vi "Host_Model_Updating.vi"(11 "Setup Parameters and Controls":T3={"Modeling Parameters input controls"={"beam_length"=0.3525, "youngs_modulus"=209500000000.0, "torsion_spring"=0.0, "beam_height"=0.00635, "beam_width"=0.0508, "beam_density"=7900.0, "number_of_FEA_nodes"=40, "accelerometer_mass"=0.055}, "Mockbear input controls"={"Dataset"="test7", "Resample Method"=enum."Auto Resample"}, "Simulation Parameters input controls"={"Eigensolver "=enum."LEMP", "Models Forcasted"=5, "Max Roller Velocity"=3.32, "Max Roller Position Percent"=0.43, "Min Roller Position Percent"=0.155}, "Program Controls"={"Frequency KF"=TRUE, "Pinned State KF"=FALSE, "FFT Bounding"=FALSE, "Filter Constants Frequency"={"Measurement Variance"=0.4, "State Variance"=0.01, "Threshold"=1000000000.0}, "Filter Constants Position"={"Measurement Variance"=0.4, "State Variance"=0.9, "Threshold"=1000000000.0}, "Moving Window Size"=10, "Time Series buffer"=10000.0, "Record Time Series Data"=FALSE, "Record Moving Window Data"=FALSE, "Record Online Error Metrics "=TRUE, "Record Statistics"=TRUE}}) -> ()   [LabVIEW 2021]
uses:
  Model_Updating_Classes/DROPBEAR_Model_Updating/DROPBEAR_Model_Updating.lvclass
panel:
  in  "Tab Control":enum32{"Time Series", "Statistics", "Controls"}(tab)
  out "Frequency":dynamicdata(graph)
  out "Meter":dynamicdata(graph)
  out "Nodal":dynamicdata(graph)
  out "DAQ Time cost":T1
  out "FFT Time cost":T1
  out "FEA Time cost":T1
  out "FFT KF Time cost":T1
  out "Sampling Time cost":T1
  out "State KF Time cost":T1
  out "Cycle Time cost":T1
  out "StatisticsTime cost":T1
  out "Signal Quality Stats Frequency":T2
  out "Signal Quality Stats Position":T2
  out "Average Cycle Time (ms)":dbl
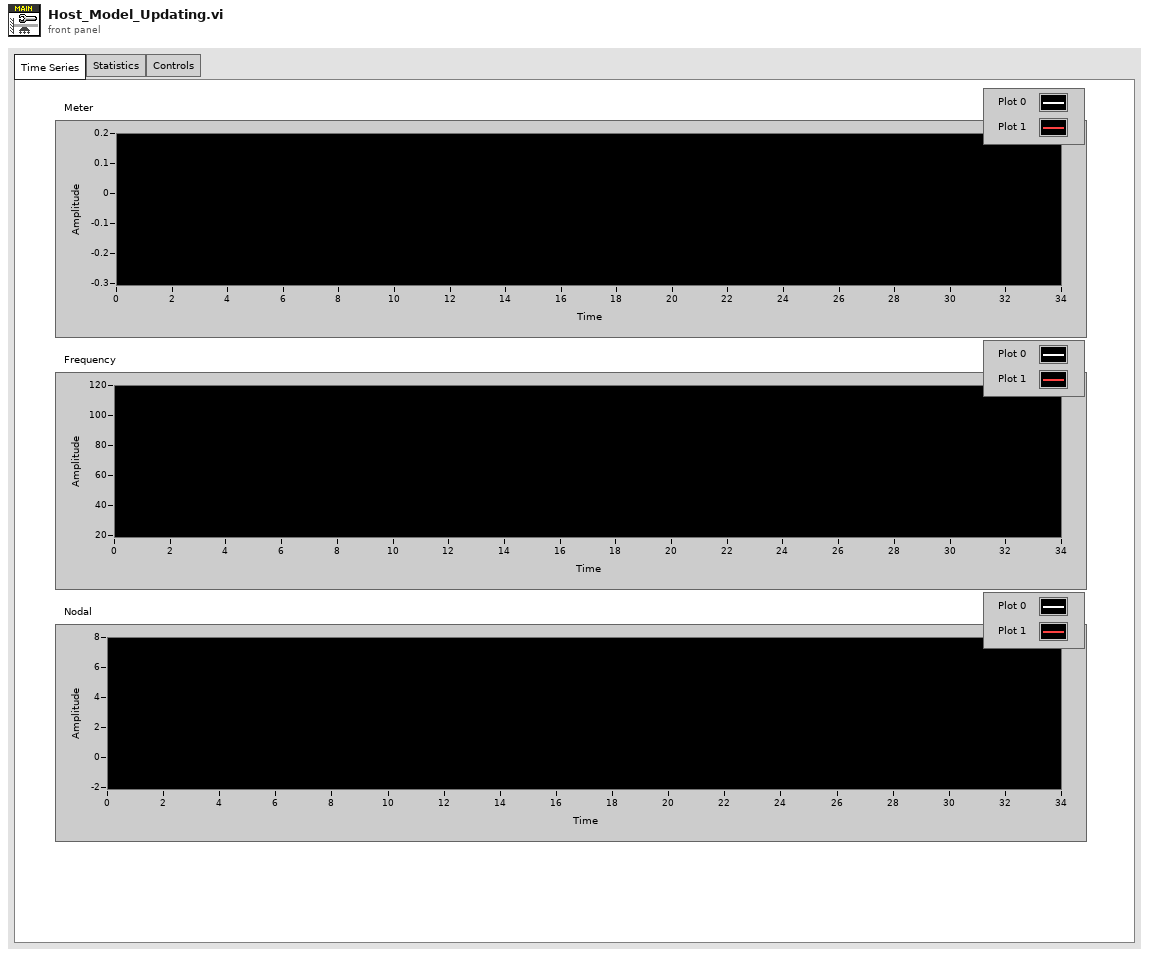
[diagram p1: front panel]
types:
  T1 = cluster{"Cumulative_mean":dbl, "Cumulative_mean_square ":dbl, "Cumulative_variance":dbl, "Max":dbl, "Min":dbl, "Number_of_samples":i32}
  T2 = cluster{"SNR":dbl, "TRAC":dbl, "Cumulative_mean":dbl, "Cumulative_mean_square ":dbl, "Cumulative_variance":dbl, "Max":dbl, "Min":dbl, "Number_of_samples":i32}
  T3 = cluster{"Modeling Parameters input controls":cluster{"beam_length":dbl, "youngs_modulus":dbl, "torsion_spring":dbl, "beam_height":dbl, "beam_width":dbl, "beam_density":dbl, "number_of_FEA_nodes":i32, "accelerometer_mass":dbl}, "Mockbear input controls":cluster{"Dataset":string, "Resample Method":enum16{"Recorded", "Auto Resample", "Custom Resample"}}, "Simulation Parameters input controls":cluster{"Eigensolver ":enum16{"LabVIEW Cholesky", "LabVIEW General", "LabVIEW Inverse", "LEMP"}, "Models Forcasted":i32, "Max Roller Velocity":dbl, "Max Roller Position Percent":dbl, "Min Roller Position Percent":dbl}, "Program Controls":cluster{"Frequency KF":bool, "Pinned State KF":bool, "FFT Bounding":bool, "Filter Constants Frequency":cluster{"Measurement Variance":dbl, "State Variance":dbl, "Threshold":dbl}, "Filter Constants Position":cluster{"Measurement Variance":dbl, "State Variance":dbl, "Threshold":dbl}, "Moving Window Size":i32, "Time Series buffer":dbl, "Record Time Series Data":bool, "Record Moving Window Data":bool, "Record Online Error Metrics ":bool, "Record Statistics":bool}}
  T4 = cluster{"Signal Quality Stats Frequency":cluster{"SNR":dbl, "TRAC":dbl, "Cumulative_mean":dbl, "Cumulative_mean_square ":dbl, "Cumulative_variance":dbl, "Max":dbl, "Min":dbl, "Number_of_samples":i32}, "Signal Quality Stats Position":cluster{"SNR":dbl, "TRAC":dbl, "Cumulative_mean":dbl, "Cumulative_mean_square ":dbl, "Cumulative_variance":dbl, "Max":dbl, "Min":dbl, "Number_of_samples":i32}}
  T5 = cluster{"DAQ Time cost":cluster{"Cumulative_mean":dbl, "Cumulative_mean_square ":dbl, "Cumulative_variance":dbl, "Max":dbl, "Min":dbl, "Number_of_samples":i32}, "FFT Time cost":cluster{"Cumulative_mean":dbl, "Cumulative_mean_square ":dbl, "Cumulative_variance":dbl, "Max":dbl, "Min":dbl, "Number_of_samples":i32}, "FFT KF Time cost":cluster{"Cumulative_mean":dbl, "Cumulative_mean_square ":dbl, "Cumulative_variance":dbl, "Max":dbl, "Min":dbl, "Number_of_samples":i32}, "Sampling Time cost":cluster{"Cumulative_mean":dbl, "Cumulative_mean_square ":dbl, "Cumulative_variance":dbl, "Max":dbl, "Min":dbl, "Number_of_samples":i32}, "FEA Time cost":cluster{"Cumulative_mean":dbl, "Cumulative_mean_square ":dbl, "Cumulative_variance":dbl, "Max":dbl, "Min":dbl, "Number_of_samples":i32}, "State KF Time cost":cluster{"Cumulative_mean":dbl, "Cumulative_mean_square ":dbl, "Cumulative_variance":dbl, "Max":dbl, "Min":dbl, "Number_of_samples":i32}, "Cycle Time cost":cluster{"Cumulative_mean":dbl, "Cumulative_mean_square ":dbl, "Cumulative_variance":dbl, "Max":dbl, "Min":dbl, "Number_of_samples":i32}, "StatisticsTime cost":cluster{"Cumulative_mean":dbl, "Cumulative_mean_square ":dbl, "Cumulative_variance":dbl, "Max":dbl, "Min":dbl, "Number_of_samples":i32}}
  T6 = cluster{"Frequency":dynamicdata, "Meters":dynamicdata, "Nodal":dynamicdata}
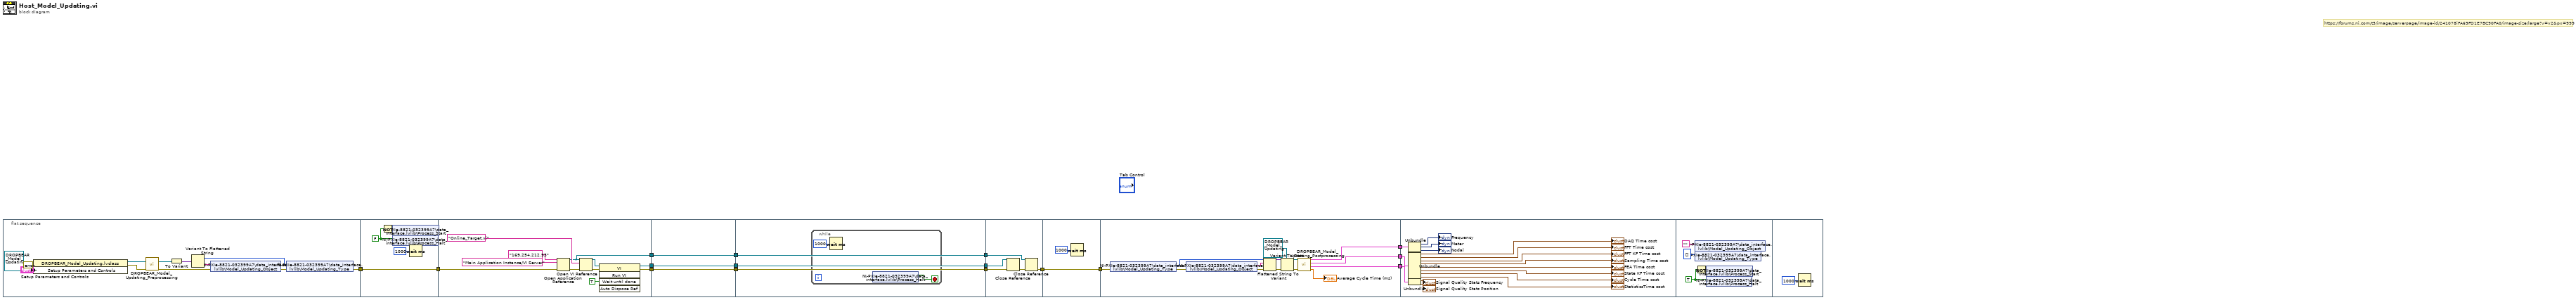
[diagram p0: block diagram]
diagram:
  # "https://forums.ni.com/t5/image/serverpage/image-id/241078iFA69FD1E7BC90FA0/image-size/large?v=v2&px=999"
  n1 = flat-sequence {
    tunnel: [w23] -> w11
    tunnel: [w32] -> w16
    tunnel: w11 -> [w32]
    tunnel: w16 -> [w37]
    tunnel: [w33] -> w9
    tunnel: [w35] -> w7
    tunnel: [w34] -> w5
    tunnel: w9 -> [w46]
    tunnel: [w46] -> w8
    tunnel: w7 -> [w45]
    tunnel: [w45] -> w6
    tunnel: w5 -> [w44]
    tunnel: [w44] -> w4
    tunnel: [w49] -> w3
    tunnel: [w48] -> w2
    tunnel: [w47] -> w1
    tunnel: w4 -> [w47]
    tunnel: w6 -> [w48]
    tunnel: w8 -> [w49]
    tunnel: w3 -> [w56]
    tunnel: [w54] -> w10
    tunnel: w2 -> [w53]
    tunnel: w1 -> [w52]
    tunnel: [w57] -> w15
    tunnel: w10 -> [w57]
    tunnel: w15 -> [w64]
    tunnel: [w61] -> w14
    tunnel: [w60] -> w13
    tunnel: [w59] -> w12
    tunnel: w12 -> [w88]
    tunnel: w13 -> [w85]
    tunnel: w14 -> [w76]
    frame #0 {
      n2 = property class="DROPBEAR_Model_Updating.lvclass"(reference=refnum<class "DROPBEAR_Model_Updating.lvclass"> refnum ("DROPBEAR_Model_Updating.lvclass"), error in=errorcluster {"status"=FALSE, "code"=0, "source"=""} ("error in (no error)"), "Setup Parameters and Controls"="Setup Parameters and Controls") -> (reference out=w22:refnum<class "DROPBEAR_Model_Updating.lvclass">, error out=w18:errorcluster)
      n3 = call-dynamic "DROPBEAR_Model_Updating_Preprocessing.vi"("error in (no error)"=w18, "DROPBEAR_Model_Updating in"=w22) -> ("error out"=w27:errorcluster, "DROPBEAR_Model_Updating out"=w28:refnum<class "DROPBEAR_Model_Updating.lvclass">)  [unwired: 8 in]
      n4 = To Variant(anything=w28) -> (Variant=w26:variant)
      n5 = Variant To Flattened String(Variant=w26) -> (data string=w25:string, 1:w17:i16[])
      n6 = shared-variable "NI-PXIe-8821-032399A7\\data_interface.lvlib\\Model_Updating_Object"(w25, error in=w27) -> (error out=w24:errorcluster)
      n7 = shared-variable "NI-PXIe-8821-032399A7\\data_interface.lvlib\\Model_Updating_Type"(w17, error in=w24) -> (error out=w23:errorcluster)
    }
    frame #1 {
      w29 = FALSE ("Process_Halt")
      n8 = Not(x=w29) -> (.not. x?=w30:bool)
      n9 = shared-variable "NI-PXIe-8821-032399A7\\data_interface.lvlib\\Process_Start"(w30) -> ()  [unwired: 1 in, 1 out]
      n10 = shared-variable "NI-PXIe-8821-032399A7\\data_interface.lvlib\\Process_Halt"(w29) -> ()  [unwired: 1 in, 1 out]
      n11 = Wait (ms)(milliseconds to wait=u32 1000) -> ()  [unwired: 1 out]
    }
    frame #2 {
      n12 = Open Application Reference(8:w37, 10:"Main Application Instance/VI Server", 11:"169.254.212.93") -> (0:w41:errorcluster, 3:w34:refnum<vi>)  [unwired: 1 in]
      n13 = Open VI Reference(application reference (local)=w34, vi path="Online_Target.vi", error in (no error)=w41) -> (vi reference=w42:refnum<vi>, error out=w43:errorcluster)  [unwired: 3 in]
      n14 = invoke class="VI" method="Run VI"(reference=w42, error in=w43, "Wait until done"=TRUE ("Wait Until Done")) -> (reference out=w35:refnum<vi>, error out=w33:errorcluster)  [unwired: 2 in, 3 out]
    }
    frame #3 {
    }
    frame #4 {
      n15 = while {
        stop <- w51 stop-if-true
        n16 = Wait (ms)(milliseconds to wait=u32 1000) -> ()  [unwired: 1 out]
        n17 = shared-variable "NI-PXIe-8821-032399A7\\data_interface.lvlib\\Process_Halt"() -> (w51:bool)  [unwired: 1 in, 1 out]
      }
    }
    frame #5 {
      n18 = Close Reference(reference=w53, error in (no error)=w56) -> (error out=w55:errorcluster)
      n19 = Close Reference(reference=w52, error in (no error)=w55) -> (error out=w54:errorcluster)
    }
    frame #6 {
      n20 = Wait (ms)(milliseconds to wait=u32 1000) -> ()  [unwired: 1 out]
    }
    frame #7 {
      n21 = shared-variable "NI-PXIe-8821-032399A7\\data_interface.lvlib\\Model_Updating_Type"(error in=w64) -> (w68:i16[], error out=w71:errorcluster)
      n22 = shared-variable "NI-PXIe-8821-032399A7\\data_interface.lvlib\\Model_Updating_Object"(error in=w71) -> (w69:string, error out=w70:errorcluster)
      n23 = Flattened String To Variant(4:w70, 6:w69, 7:w68) -> (0:w65:errorcluster, 3:w66:variant)
      n24 = Variant To Data(error in=w65, type=refnum<class "DROPBEAR_Model_Updating.lvclass"> refnum ("DROPBEAR_Model_Updating.lvclass"), Variant=w66) -> (data=w63:refnum<class "DROPBEAR_Model_Updating.lvclass">, error out=w62:errorcluster)
      n25 = call "DROPBEAR_Model_Updating_Postprocessing.vi"("error in (no error)"=w62, "DROPBEAR_Model_Updating in"=w63) -> ("Cycle time (ms)"=→"Average Cycle Time (ms)":dbl, "Signal Quality"=w59:T4, "Timing stats"=w60:T5, "Plots"=w61:T6)  [unwired: 6 in]
    }
    frame #8 {
      n26 = Unbundle(w76) -> ("Frequency"=→"Frequency":dynamicdata, "Meters"=→"Meter":dynamicdata, "Nodal"=→"Nodal":dynamicdata)
      n27 = Unbundle(w85) -> ("DAQ Time cost"=→"DAQ Time cost":T1, "FFT Time cost"=→"FFT Time cost":T1, "FFT KF Time cost"=→"FFT KF Time cost":T1, "Sampling Time cost"=→"Sampling Time cost":T1, "FEA Time cost"=→"FEA Time cost":T1, "State KF Time cost"=→"State KF Time cost":T1, "Cycle Time cost"=→"Cycle Time cost":T1, "StatisticsTime cost"=→"StatisticsTime cost":T1)
      n28 = Unbundle(w88) -> ("Signal Quality Stats Frequency"=→"Signal Quality Stats Frequency":T2, "Signal Quality Stats Position"=→"Signal Quality Stats Position":T2)
    }
    frame #9 {
      w90 = TRUE ("Process_Halt")
      n29 = shared-variable "NI-PXIe-8821-032399A7\\data_interface.lvlib\\Model_Updating_Object"("") -> ()  [unwired: 1 in, 1 out]
      n30 = shared-variable "NI-PXIe-8821-032399A7\\data_interface.lvlib\\Model_Updating_Type"(i16[] [] ("Model_Updating_Type")) -> ()  [unwired: 1 in, 1 out]
      n31 = Not(x=w90) -> (.not. x?=w89:bool)
      n32 = shared-variable "NI-PXIe-8821-032399A7\\data_interface.lvlib\\Process_Start"(w89) -> ()  [unwired: 1 in, 1 out]
      n33 = shared-variable "NI-PXIe-8821-032399A7\\data_interface.lvlib\\Process_Halt"(w90) -> ()  [unwired: 1 in, 1 out]
    }
    frame #10 {
      n34 = Wait (ms)(milliseconds to wait=u32 1000) -> ()  [unwired: 1 out]
    }
  }
